vi "Auto Number Get Next MSN.vi"(8 "error in (no error)":errorcluster, 11 "Connection Refnum":T1) -> (0 "error out":errorcluster, 2 "Model Number":string, 3 "Connection Refnum":T1)   [LabVIEW 2011]
uses:
  SI.LIB/ODBC/SQL Controls/Connection Refnum.ctl
  Auto Number Record.ctl
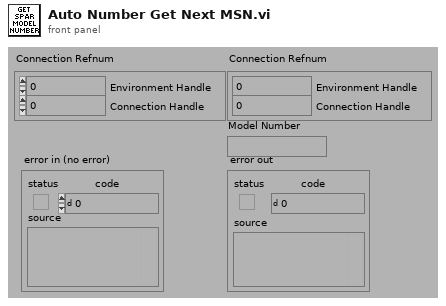
[diagram p1: front panel]
types:
  T1 = typedef "Connection Refnum.ctl" = cluster{"Environment Handle":i32, "Connection Handle":i32}
  T2 = typedef "Auto Number Record.ctl" = cluster{"ixAutoNumber":i32, "sModelNumber":string, "sSerialNumber":string}
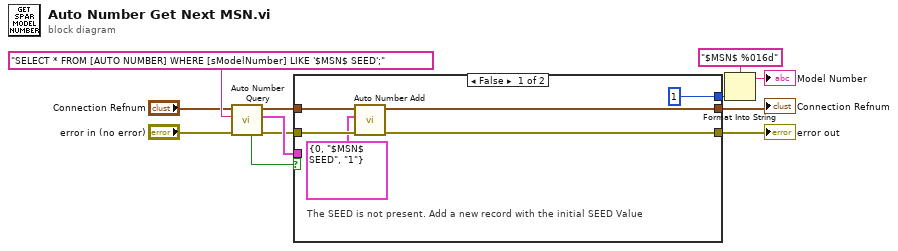
[diagram p0: block diagram]
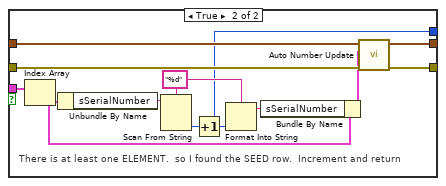
[diagram p2: hidden frame]
diagram:
  n1 = call "Auto Number Query.vi"("error in (no error)"="error in (no error)", "Query"="SELECT * FROM [AUTO NUMBER] WHERE [sModelNumber] LIKE '$MSN$ SEED';", "Connection Refnum"="Connection Refnum") -> ("error out"=w8:errorcluster, "Auto Number Records"=w10:T2[], "Connection Refnum"=w9:T1, "Data Present?"=w11:bool)  [unwired: 5 out]
  n2 = case shown="False" w11 {
    tunnel: w10 -> [_ w30]
    tunnel: w9 -> [w16 w28]
    tunnel: w8 -> [w15 w27]
    tunnel: [w17 w26] -> w3
    tunnel: [w18 w25] -> w4
    tunnel: [1 w22] -> w6
    frame False {
      # "The SEED is not present. Add a new record with the initial SEED Value"
      n3 = call "Auto Number Add.vi"("error in (no error)"=w15, "Auto Number Record"=T2 {"ixAutoNumber"=0, "sModelNumber"="$MSN$ SEED", "sSerialNumber"="1"} ("Auto_Number Record"), "Connection Refnum"=w16) -> ("error out"=w17:errorcluster, "Connection Refnum"=w18:T1)  [unwired: 7 out]
    }
    frame True {
      w23 = "%d" ("format string")
      # "There is at least one ELEMENT.  so I found the SEED row.  Increment and return"
      n4 = Index Array(array=w30) -> (element=w19:T2)  [unwired: 1 in]
      n5 = Unbundle By Name(w19) -> ("sSerialNumber"=w21:string)
      n6 = Scan From String(format string=w23, input string=w21) -> (output 1=w29:i32)  [unwired: 2 in, 4 out]
      n7 = Increment(x=w29) -> (x+1=w22:i32)
      n8 = Format Into String(format string=w23, w22) -> (resulting string=w20:string)  [unwired: 2 in, 1 out]
      n9 = Bundle By Name(cluster=w19, "sSerialNumber"=w20) -> (w24:T2)
      n10 = call "Auto Number Update.vi"("error in (no error)"=w27, "Auto Number Record"=w24, "Connection Refnum"=w28) -> ("error out"=w26:errorcluster, "Connection Refnum"=w25:T1)  [unwired: 7 out]
    }
  }
  "error out" <- w3
  "Connection Refnum" <- w4
  n11 = Format Into String(format string="$MSN$ %016d", w6) -> (resulting string=→"Model Number":string)  [unwired: 2 in, 1 out]
